vi "Raspberry.vi"() -> ()   [LabVIEW 2016]
panel:
  out "error out":errorcluster
  in  "ON/OFF":bool
  out "bytes written":i32
  out "Data from Raspberry":string
  in  "stop":bool
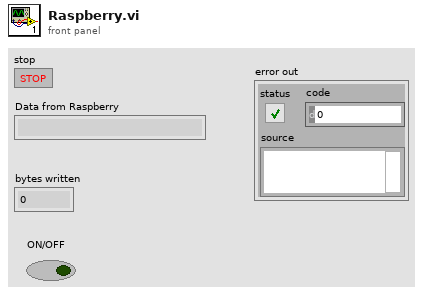
[diagram p1: front panel]
types:
  T1 = enum16{"Standard", "Buffered", "CRLF", "Immediate"}
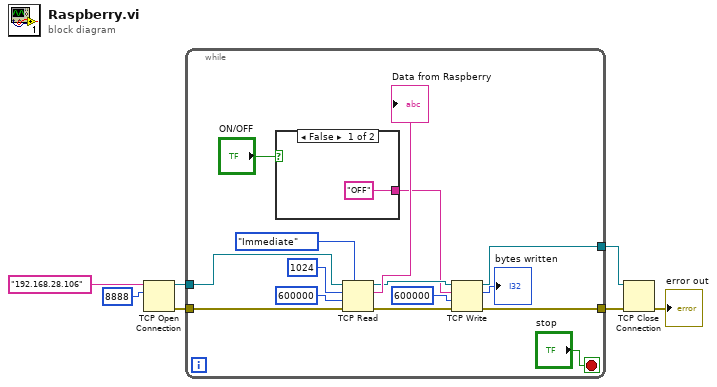
[diagram p0: block diagram]
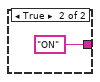
[diagram p2: hidden frame]
diagram:
  n1 = TCP Open Connection(address="192.168.28.106", remote port or service name=u16 8888) -> (connection ID=w4:refnum<k5>, error out=w5:errorcluster)  [unwired: 3 in]
  n2 = while {
    tunnel: w5 -> [w21]
    tunnel: w4 -> [w20]
    tunnel: [w14] -> w3
    tunnel: [w12] -> w2
    stop <- "stop" stop-if-true
    n3 = case shown="False" "ON/OFF" {
      tunnel: ["OFF" ("data in") "ON" ("data in")] -> w9
      frame False {
      }
      frame True {
      }
    }
    n4 = TCP Read(connection ID=w20, bytes to read=1024, error in (no error)=w21, 7:T1."Immediate" ("mode (standard)"), 9:600000 ("timeout ms (25000)")) -> (connection ID out=w13:refnum<k5>, data out=→"Data from Raspberry":string, error out=w15:errorcluster)
    n5 = TCP Write(connection ID=w13, data in=w9, error in (no error)=w15, 9:600000 ("timeout ms (25000)")) -> (connection ID out=w12:refnum<k5>, bytes written=→"bytes written":i32, error out=w14:errorcluster)
  }
  n6 = TCP Close Connection(connection ID=w2, error in (no error)=w3) -> (error out=→"error out":errorcluster)  [unwired: 1 in, 1 out]
